vi "Fall2016SemesterPIDController.vi"(0 "Encoder Angle (degrees)":dbl format="%.2f", 1 "Encoder Angle Setpoint (degrees)":dbl format="%.2f", 2 "PID gains":T1={"proportional gain (Kc)"=0.04, "integral time (Ti, min)"=0.0, "derivative time (Td, min)"=0.004} {"derivative time (Td, min)" min=-0.1 max=0.1 step=1e-05 format="%.5f"; "integral time (Ti, min)" min=-10.0 max=10.0 step=1e-05 format="%.5f"; "proportional gain (Kc)" format="%.3f"}, 4 "Old Error":dbl) -> (5 "New Error":dbl, 7 "SpinFraction":dbl)   [LabVIEW 2018]
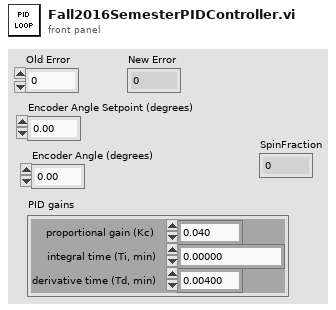
[diagram p1: front panel]
types:
  T1 = cluster{"proportional gain (Kc)":dbl, "integral time (Ti, min)":dbl, "derivative time (Td, min)":dbl}
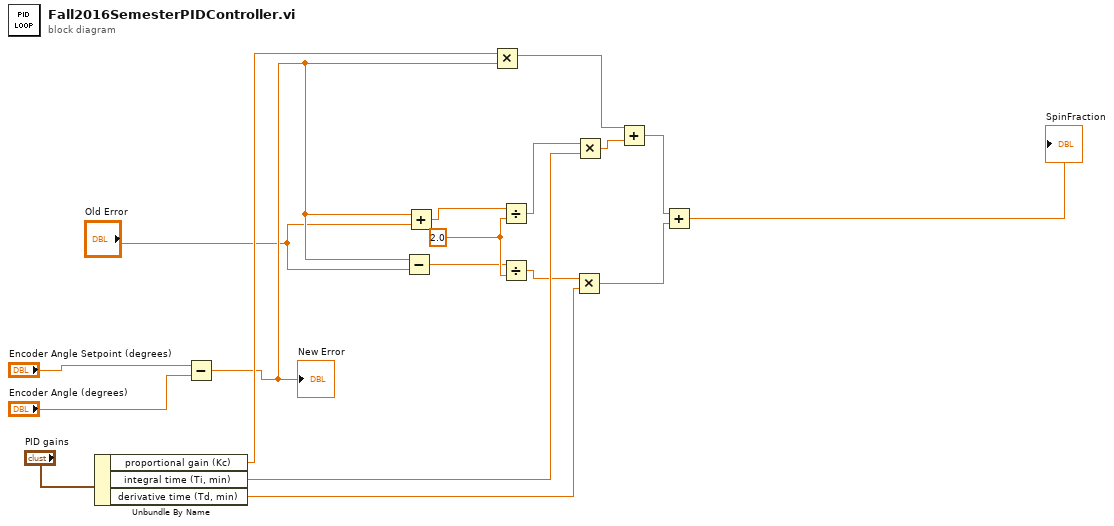
[diagram p0: block diagram]
diagram:
  w11 = 2.0 ("y")
  n1 = Unbundle By Name("PID gains") -> ("proportional gain (Kc)"=w15:dbl, "integral time (Ti, min)"=w13:dbl, "derivative time (Td, min)"=w12:dbl)
  n2 = Subtract(x="Encoder Angle Setpoint (degrees)", y="Encoder Angle (degrees)") -> (x-y=w14:dbl)
  "New Error" <- w14
  n3 = Subtract(x=w14, y="Old Error") -> (x-y=w10:dbl)
  n4 = Add(x=w14, y="Old Error") -> (x+y=w9:dbl)
  n5 = Multiply(x=w15, y=w14) -> (x*y=w6:dbl)
  n6 = Divide(x=w9, y=w11) -> (x/y=w7:dbl)
  n7 = Divide(x=w10, y=w11) -> (x/y=w8:dbl)
  n8 = Multiply(x=w8, y=w12) -> (x*y=w3:dbl)
  n9 = Multiply(x=w7, y=w13) -> (x*y=w5:dbl)
  n10 = Add(x=w6, y=w5) -> (x+y=w4:dbl)
  n11 = Add(x=w4, y=w3) -> (x+y=→"SpinFraction":dbl)
